vi "Read Conversion Time.vi"(8 "error in":errorcluster, 11 "NI 9224 in":refnum<class "NI 9224.lvclass">) -> (0 "error out":errorcluster, 2 "conversion time":T1, 3 "NI 9224 out":refnum<class "NI 9224.lvclass">)   [LabVIEW 2020, in "Scan Engine Scripting.lvlib" / "NI 9224.lvclass"]
uses:
  NI 9224.lvclass
  Utility/Shared Properties/Conversion Time.ctl
  NI 9224.lvclass/NI 9224.ctl
  Scan Engine Scripting.lvlib
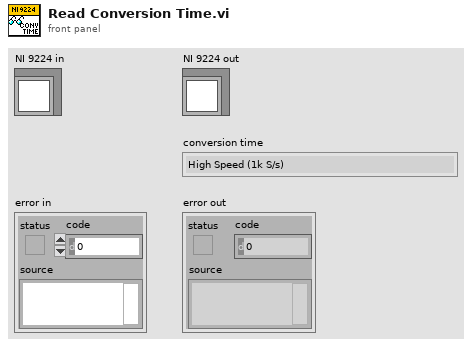
[diagram p1: front panel]
types:
  T1 = typedef "Scan Engine Scripting.lvlib/Conversion Time.ctl" = enum16{"High Speed (1k S/s)", "Medium Speed (100 S/s)", "Medium Resolution (50/60Hz Rejection - 12 S/s)", "High Resolution (50/60Hz Rejection - 2 S/s)"}
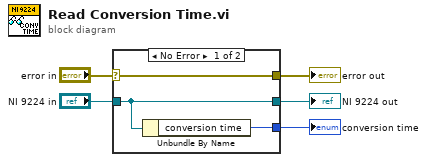
[diagram p0: block diagram]
diagram:
  n1 = case shown="No Error" "error in" {
    selector: "error in" -> [w8 w9]
    tunnel: [w8 w9] -> w4
    tunnel: [w7 w10] -> w2
    tunnel: "NI 9224 in" -> [w7 w10]
    tunnel: [w6 _] -> w1
    frame No Error {
      n2 = Unbundle By Name(w7) -> ("conversion time"=w6:T1)
    }
    frame Error {
    }
  }
  "error out" <- w4
  "NI 9224 out" <- w2
  "conversion time" <- w1
